vi "CreateDO.vi"(0 "Sig_DI_Simple in":refnum<class "DO.lvclass">, 5 "error in (no error)":errorcluster, 12 "Tags":T1, 13 "Logger":refnum<class "Logger.lvclass">) -> (14 "Sig_DI_Simple out":refnum<class "DO.lvclass">, 19 "error out":errorcluster)   [LabVIEW 2019, in "DO.lvclass"]
uses:
  DO.lvclass
  D:/GIT H4000/H4000/src/Signal_class/Signal.lvclass
  Proccess_class/TAGs.ctl
  Logger_class/Logger.lvclass
  Signal_class/Signal.lvclass
  Proccess_class/Proccess.lvclass
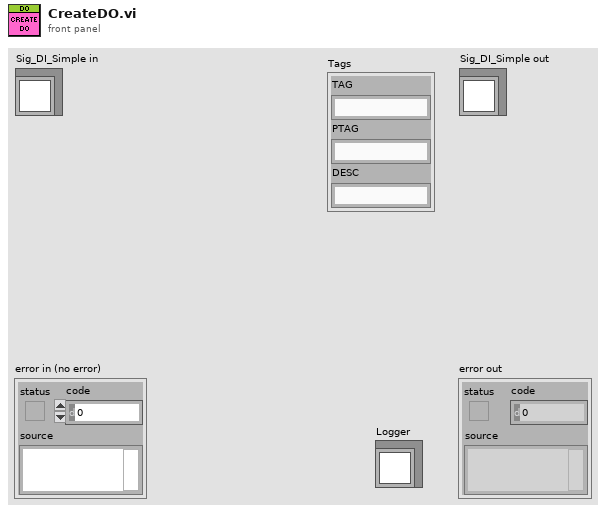
[diagram p1: front panel]
types:
  T1 = typedef "Proccess.lvclass/TAGs.ctl" = cluster{"TAG":string, "PTAG":string, "DESC":string}
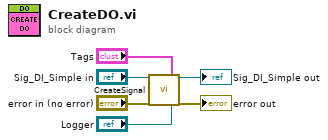
[diagram p0: block diagram]
diagram:
  n1 = call "CreateSignal.vi"("Signal in"="Sig_DI_Simple in", "error in (no error)"="error in (no error)", "Tags"="Tags", "Logger"="Logger") -> ("Signal out"=→"Sig_DI_Simple out":refnum<class "DO.lvclass">, "error out"=→"error out":errorcluster)  [unwired: 14 in]
